vi "Get Lens Mode.vi"() -> ()   [LabVIEW 2011]
uses:
  SesWrapper/SesWrapper.lvlib
panel:
  in  "Element Set":string="Low Pass (UPS)"
  in  "Working Directory":string="D:\\SES 1.2.6-r6"
  in  "Instrument Configuration File":string="D:\\SES 1.2.6-r6\\data\\4ES288WALInstrument.dat"
  out "Pass Energy":dbl
  out "size out":i32
  out "Current Lens Mode":string
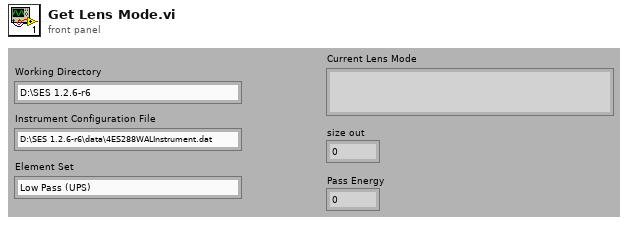
[diagram p1: front panel]
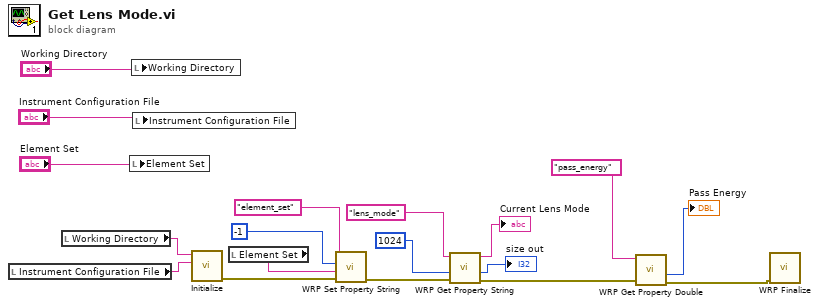
[diagram p0: block diagram]
diagram:
  n1 = local read "Instrument Configuration File"() -> (w6:string)
  n2 = local read "Working Directory"() -> (w7:string)
  n3 = local write "Element Set"("Element Set") -> ()
  n4 = local write "Working Directory"("Working Directory") -> ()
  n5 = local write "Instrument Configuration File"("Instrument Configuration File") -> ()
  n6 = call "Initialize.vi"("Instrument Configuration File"=w6, "working_directory"=w7) -> ("error out"=w3:errorcluster)  [unwired: 9 in]
  n7 = local read "Element Set"() -> (w4:string)
  n8 = call "WRP Set Property String.vi"("error in (no error)"=w3, "value"=w4, "index"=-1, "property"="element_set") -> ("error out"=w2:errorcluster)  [unwired: 6 in, 1 out]
  n9 = call "WRP Get Property String.vi"("error in (no error)"=w2, "size"=1024, "property"="lens_mode") -> ("error out"=w14:errorcluster, "size out"=→"size out":i32, "value"=→"Current Lens Mode":string)  [unwired: 5 in, 1 out]
  n10 = call "WRP Get Property Double.vi"("error in (no error)"=w14, "property"="pass_energy") -> ("error out"=w13:errorcluster, "size out"=→"Pass Energy":i32)  [unwired: 6 in, 2 out]
  n11 = call "WRP Finalize.vi"("error in (no error)"=w13) -> ()  [unwired: 9 in, 2 out]
